vi "Configure Waveform Characteristics(Shape).vi"(0 "VISA resource name":refnum<visa-resource-name>, 5 "Output Channel (1: Channel 1)":i32(ring)=1 items=["Channel 1"=1, "Channel 2"=2], 9 "Waveform Shape (0: Sinusoid)":i32(ring) items=["Sinusoid", "Square", "Ramp", "Pulse", "Noise", "User", "Harmonic", "Custom", "DC", "AbsSine", "AbsSineHalf", "AmpALT", "AttALT", "GaussPulse", "NegRamp", "NPulse", "PPulse", "SineTra", "SineVer", "StairDn", "StairUD", "StairUp", "Trapezia", "BandLimited", "Butterworth", "Chebyshev1", "Chebyshev2", "Combin", "CPulse", "CWPulse", "DampedOsc", "DualTone", "Gamma", "GateVibr", "LEMPulse", "MCNoise", "Discharge", "Pahcur", "Quake", "Radar", "Ripple", "RoundHalf", "RoundPM", "StepResp", "SwingOsc", "TV", "Voice", "AM", "FM", "PM", "PWM", "PFM", "Cardiac", "EOG", "EEG", "EMG", "Pulseilogram", "ResSpeed", "LFPulse", "Tens1", "Tens2", "Tens3", "Lgnition", "ISO16750-2 SP", "ISO16750-2 VR", "ISO7637-2 TP1", "ISO7637-2 TP2A", "ISO7637-2 TP2B", "ISO7637-2 TP3A", "ISO7637-2 TP3B", "ISO7637-2 TP4", "ISO7637-2 TP5A", "ISO7637-2 TP5B", "SCR", "Surge", "Airy", "Besselj", "Bessely", "Cauchy", "Cubic", "Dirichlet", "Erf", "Erfc", "Erfclnv", "Erflnv", "ExpFall", "ExpRise", "Gauss", "HaverSine", "Laguerre", "Laplace", "Legend", "Log", "LogNormal", "Lorentz", "Maxwell", "Rayleigh", "Versiera", "Weibull", "ARB_X2", "CosH", "CosInt", "Cot", "CotHCon", "CotHPro", "CscCon", "CscPro", "CscHCon", "CscHPro", "RecipCon", "RecipPro", "SecCon", "SecPro", "SecH", "Sinc", "SinH", "SinInt", "Sqrt", "Tan", "TanH", "ACos", "ACosH", "ACotCon", "ACotPro", "ACotHCon", "ACotHPro", "ACscCon", "ACscPro", "ACscHCon", "ACscHPro", "ASecCon", "ASsePro", "ASecH", "ASin", "ASinH", "ATan", "ATanH", "Barlett", "BarthannWin", "Blackman", "BlackmanH", "BlackmanWin", "Boxcar", "ChebWin", "FlattopWin", "Hamming", "Hanning", "Kaiser", "NuttallWin", "ParzenWin", "TaylorWin", "Triang", "TukeyWin"], 11 "error in (no error)":errorcluster) -> (4 "VISA resource name out":refnum<visa-resource-name>, 15 "error out":errorcluster)   [LabVIEW 2012, in "RIGOL DG4000 Series.lvlib"]
doc: "Configures the waveform shape.\n\nNotes:\n(1)This VI selects the output waveform of the instrument when Mod, Sweep and Burst are disabled.\n(2)This VI selects the carrier waveform corresponding to the function when Mod, Sweep or Burst is currently enabled."
uses:
  <instrlib>/RIGOL DG4000 Series/RIGOL DG4000 Series.lvlib
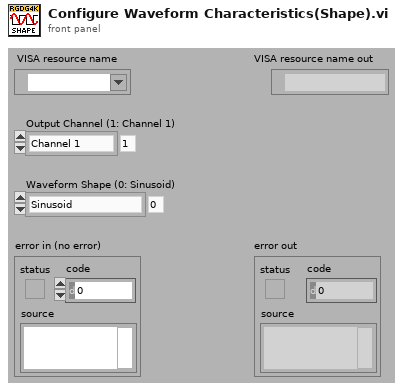
[diagram p1: front panel]
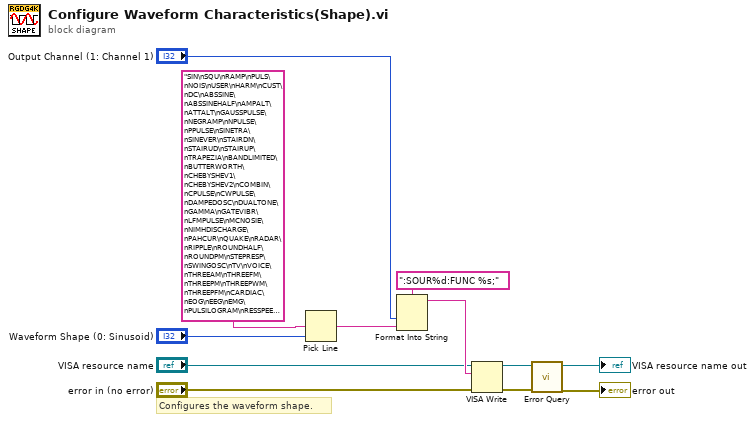
[diagram p0: block diagram]
diagram:
  # "Configures the waveform shape."
  n1 = Pick Line(multi-line string="SIN\nSQU\nRAMP\nPULS\nNOIS\nUSER\nHARM\nCUST\nDC\nABSSINE\nABSSINEHALF\nAMPALT\nATTALT\nGAUSSPULSE\nNEGRAMP\nNPULSE\nPPULSE\nSINETRA\nSINEVER\nSTAIRDN\nSTAIRUD\nSTAIRUP\nTRAPEZIA\nBANDLIMITED\nBUTTERWORTH\nCHEBYSHEV1\nCHEBYSHEV2\nCOMBIN\nCPULSE\nCWPULSE\nDAMPEDOSC\nDUALTONE\nGAMMA\nGATEVIBR\nLFMPULSE\nMCNOSIE\nNIMHDISCHARGE\nPAHCUR\nQUAKE\nRADAR\nRIPPLE\nROUNDHALF\nROUNDPM\nSTEPRESP\nSWINGOSC\nTV\nVOICE\nTHREEAM\nTHREEFM\nTHREEPM\nTHREEPWM\nTHREEPFM\nCARDIAC\nEOG\nEEG\nEMG\nPULSILOGRAM\nRESSPEED\nLFPULSE\nTENS1\nTENS2\nTENS3\nIGNITION\nISO167502SP\nISO167502VR\nISO76372TP1\nISO76372TP2A\nISO76372TP2B\nISO76372TP3A\nISO76372TP3B\nISO76372TP4\nISO76372TP5A\nISO76372TP5B\nSCR\nSURGE\nAIRY\nBESSELJ\nBESSELY\nCAUCHY\nCUBIC\nDIRICHLET\nERF\nERFC\nERFCINV\nERFINV\nEXPFALL\nEXPRISE\nGAUSS\nHAVERSINE\nLAGUERRE\nLAPLACE\nLEGEND\nLOG\nLOGNORMAL\nLORENTZ\nMAXWELL\nRAYLEIGH\nVERSIERA\nWEIBULL\nX2DATA\nCOSH\nCOSINT\nCOT\nCOTHCON\nCOTHPRO\nCSCCON\nCSCPRO\nCSCHCON\nCSCHPRO\nRECIPCON\nRECIPPRO\nSECCON\nSECPRO\nSECH\nSINC\nSINH\nSININT\nSQRT\nTAN\nTANH\nACOS\nACOSH\nACOTCON\nACOTPRO\nACOTHCON\nACOTHPRO\nACSCCON\nACSCPRO\nACSCHCON\nACSCHPRO\nASECCON\nASECPRO\nASECH\nASIN\nASINH\nATAN\nATANH\nBARLETT\nBARTHANN\nBLACKMAN\nBLACKMANH\nBOHMANWIN\nBOXCAR\nCHEBWIN\nFLATTOPWIN\nHAMMING\nHANNING\nKAISER\nNUTTALLWIN\nPARZENWIN\nTAYLORWIN\nTRIANG\nTUKEYWIN", line index="Waveform Shape (0: Sinusoid)") -> (output string=w8:string)  [unwired: 1 out]
  n2 = Format Into String(format string=":SOUR%d:FUNC %s;", "Output Channel (1: Channel 1)", w8) -> (resulting string=w7:string)  [unwired: 2 in, 1 out]
  n3 = VISA Write(VISA resource name="VISA resource name", write buffer=w7, error in (no error)="error in (no error)") -> (VISA resource name out=w4:refnum<visa-resource-name>, error out=w3:errorcluster)  [unwired: 1 out]
  n4 = call <instrlib>:"Error Query.vi"("error in (no error)"=w3, "VISA resource name"=w4) -> ("error out"=→"error out":errorcluster, "VISA resource name out"=→"VISA resource name out":refnum<visa-resource-name>)  [unwired: 8 out]
